vi "Read Tags.vi"(8 "error in (no error)":errorcluster, 11 "FeedItem.lvclass in":refnum<class "FeedItem.lvclass">) -> (0 "error out":errorcluster, 2 "Tags":string[](array[string]), 3 "FeedItem.lvclass out":refnum<class "FeedItem.lvclass">)   [LabVIEW 2020, in "FeedItem.lvclass"]
uses:
  <vilib>/NI_RSS/FeedItem/FeedItem.lvclass
  <vilib>/NI_RSS/FeedItem/FeedItem.lvclass/FeedItem.ctl
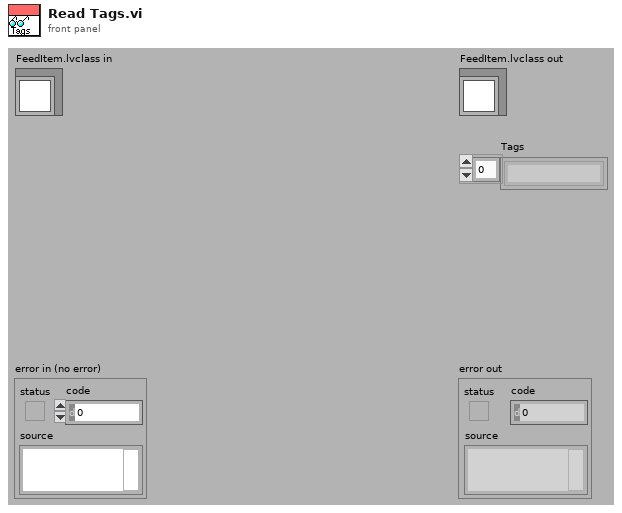
[diagram p1: front panel]
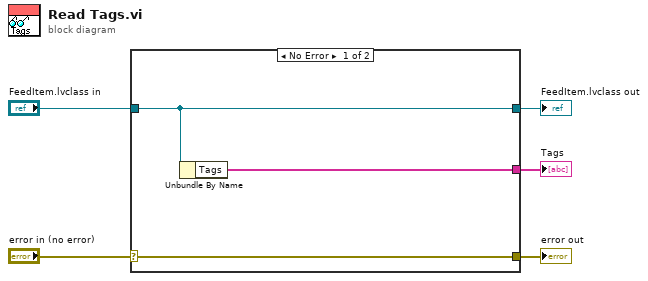
[diagram p0: block diagram]
diagram:
  n1 = case shown="No Error" "error in (no error)" {
    selector: "error in (no error)" -> [w8 w9]
    tunnel: [w8 w9] -> w4
    tunnel: [w7 w10] -> w2
    tunnel: "FeedItem.lvclass in" -> [w7 w10]
    tunnel: [w6 _] -> w1
    frame No Error {
      n2 = Unbundle By Name(w7) -> ("Tags"=w6:string[])
    }
    frame Error {
    }
  }
  "error out" <- w4
  "FeedItem.lvclass out" <- w2
  "Tags" <- w1
